vi "testir.vi"() -> ()   [LabVIEW 2019]
panel:
  out "A/AI1 (Pin 5)":dbl
  out "公分":dbl(slide) scale=0.0..200.0
  in  "stop":bool
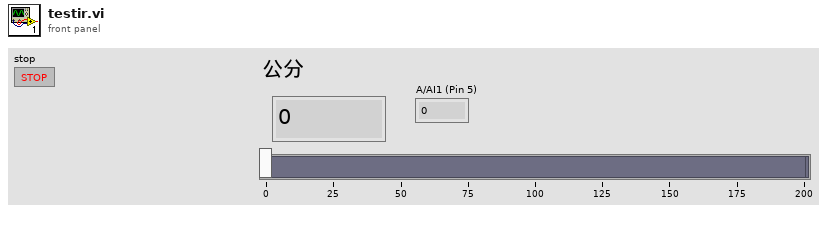
[diagram p1: front panel]
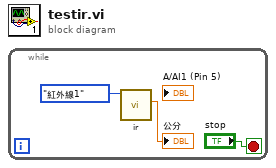
[diagram p0: block diagram]
diagram:
  n1 = while {
    stop <- "stop" stop-if-true
    n2 = call "ir.vi"("選擇紅外線"=enum16{"請選擇紅外線", "紅外線1", "紅外線2", "紅外線3", "紅外線4"}."紅外線1") -> ("公分"=→"公分":dbl)  [unwired: 9 in, 1 out]
  }
